vi "DAC8552 Example.vi"() -> ()   [LabVIEW 2020]
uses:
  <vilib>/MakerHub/LINX/Public/Peripherals/SPI/SPI CS Config.ctl
  <vilib>/MakerHub/LINX/Private/Type Defs/Peripherals/SPI/SPI CS Logic Level.ctl
  <vilib>/MakerHub/LINX/Private/Type Defs/Peripherals/SPI/SPI Configuration.ctl
  <vilib>/MakerHub/LINX/Private/Type Defs/Peripherals/SPI/SPI Bit Order.ctl
  <vilib>/MakerHub/LINX/Private/Type Defs/Peripherals/SPI/SPI Mode.ctl
  LINX-DAC8552/Power Down Mode.ctl
  LINX-DAC8552/Channel Select.ctl
  <vilib>/MakerHub/LINX/Public/Utilities/Open Local.vi
  LINX SPI/LINX SPI.lvclass
  <vilib>/MakerHub/LINX/LMH-LINX.lvlib
  LINX-DAC8552/LINX-DAC8552.lvclass
panel:
  in  "DAC B":dbl
  in  "DAC A":dbl
  in  "stop":bool
  out "Error Out":errorcluster
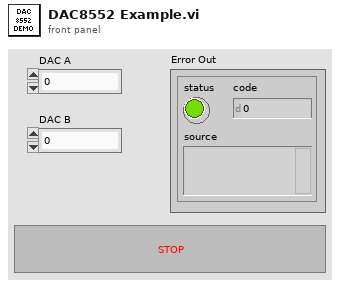
[diagram p1: front panel]
types:
  T1 = typedef "LINX-DAC8552.lvclass/Power Down Mode.ctl" = enum8{"On - Normal Operation", "Off - 1kOhm", "Off - 100kOhm", "Off - High Impedence"}
  T2 = typedef "LINX-DAC8552.lvclass/Channel Select.ctl" = enum8{"DAC A", "DAC B", "Both"}
  T3 = typedef "LMH-LINX.lvlib/SPI Configuration.ctl" = cluster{"Clock Frequency":u32, "Bit Order":T4, "SPI Mode":T5}
  T4 = typedef "LMH-LINX.lvlib/SPI Bit Order.ctl" = enum8{"LSb First", "MSb First"}
  T5 = typedef "LMH-LINX.lvlib/SPI Mode.ctl" = enum8{"Mode 0", "Mode 1", "Mode 2", "Mode 3"}
  T6 = typedef "LMH-LINX.lvlib/SPI CS Config.ctl" = cluster{"CS Channel":u8, "CS Logic Level":T7}
  T7 = typedef "LMH-LINX.lvlib/SPI CS Logic Level.ctl" = enum8{"Active Low", "Active High"}
  T8 = typedef "LMH-LINX.lvlib/LINX Ref.ctl" = cluster{"IO":T9, "Interface":T10, "LINX Device Config":T11}
  T9 = typedef "LMH-LINX.lvlib/Platform.ctl" = enum16{"Remote", "Local"}
  T10 = typedef "LMH-LINX.lvlib/Interface.ctl" = enum16{"Serial", "TCP"}
  T11 = typedef "LMH-LINX.lvlib/Device.lvlib/LINX Device Config.ctl" = cluster{"Interface":T10, "COM Port":refnum<visa-resource-name>, "TCP Configuration":T12, "Device Family":u8, "Device ID":u8, "Device Name":string, "TCP Ref":refnum<k5>, "Channels":T13}
  T12 = typedef "LMH-LINX.lvlib/Device.lvlib/TCP Config.ctl" = cluster{"IP Address":string, "Port":u16}
  T13 = typedef "LMH-LINX.lvlib/Channels.ctl" = cluster{"DI":u8[], "DO":u8[], "AI":u8[], "AO":u8[], "PWM":u8[], "QE":u8[], "UART":u8[], "I2C 2":u8[], "SPI":u8[], "CAN":u8[], "Servo":u8[], "AI Ref (V)":dbl, "AI Resolution (Bits)":u8, "AO Ref (V)":dbl, "AO Resolution (Bits)":u8}
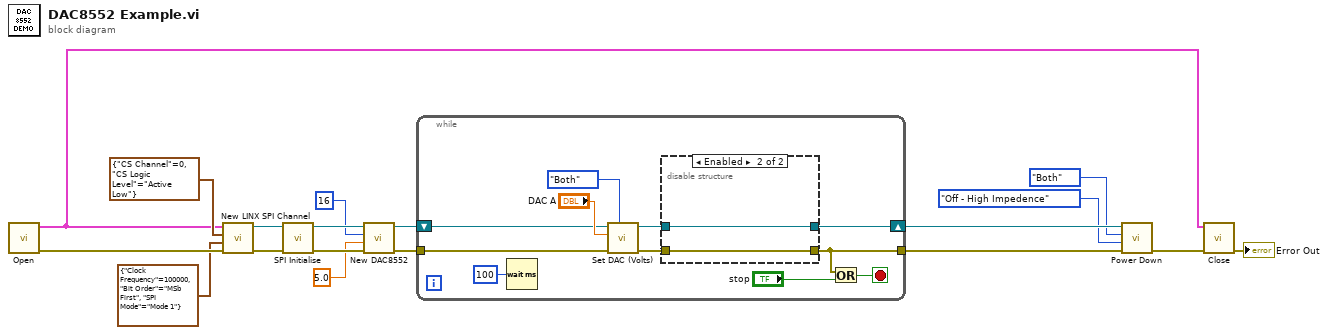
[diagram p0: block diagram]
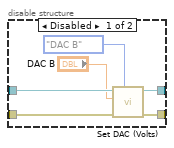
[diagram p2: hidden frame]
diagram:
  n1 = call-poly <vilib>:"Open.vi"() -> ("Error Out"=w17:errorcluster, "LINX Resource"=w13:T8)  [unwired: 9 in, 1 out]
  n2 = call "New LINX SPI Channel.vi"("error in (no error)"=w17, "SPI Configuration"=T3 {"Clock Frequency"=100000, "Bit Order"=enum."MSb First", "SPI Mode"=enum."Mode 1"}, "CS Configuration"=T6 {"CS Channel"=0, "CS Logic Level"=enum."Active Low"}, "LINX Resource"=w13) -> ("error out"=w14:errorcluster, "LINX SPI out"=w15:refnum<class "LINX SPI.lvclass">)  [unwired: 6 in]
  n3 = call-dynamic "SPI Initialise.vi"("error in (no error)"=w14, "LINX SPI in"=w15) -> ("error out"=w11:errorcluster, "LINX SPI out"=w10:refnum<class "LINX SPI.lvclass">)  [unwired: 8 in]
  n4 = call "New DAC8552.vi"("error in (no error)"=w11, "VRef (5V)"=5.0, "SPI CS Line"=u8 16, "SPI in"=w10) -> ("error out"=w6:errorcluster, "LINX-DAC8552 out"=w7:refnum<class "LINX-DAC8552.lvclass">)  [unwired: 6 in]
  n5 = while {
    tunnel: w6 -> [w26]
    shift-right: [w24] -> w3
    shift-left: w7 -> [w20]
    tunnel: [w25] -> w5
    stop <- w28 stop-if-true
    n6 = Wait (ms)(milliseconds to wait=u32 100) -> ()  [unwired: 1 out]
    n7 = call "Set DAC (Volts).vi"("Channel Select"=Channel_Select."Both", "error in (no error)"=w26, "DAC Output (V)"="DAC A", "DAC8552 in"=w20) -> ("error out"=w22:errorcluster, "DAC8552 out"=w23:refnum<class "LINX-DAC8552.lvclass">)  [unwired: 6 in]
    n8 = disable-structure shown="Enabled" {
      disable-tunnel: [w35 w36] -> w25
      disable-tunnel: [w34 w37] -> w24
      disable-tunnel: w23 -> [w33 w37]
      disable-tunnel: w22 -> [w32 w36]
      frame Disabled {
        n9 = call "Set DAC (Volts).vi"("Channel Select"=Channel_Select."DAC B", "error in (no error)"=w32, "DAC Output (V)"="DAC B", "DAC8552 in"=w33) -> ("error out"=w35:errorcluster, "DAC8552 out"=w34:refnum<class "LINX-DAC8552.lvclass">)  [unwired: 6 in]
      }
      frame Enabled {
      }
    }
    n10 = Or(x=w25, y="stop") -> (x .or. y?=w28:bool)
  }
  n11 = call "Power Down.vi"("error in (no error)"=w5, "Power Down Mode"=Power_Down_Mode."Off - High Impedence", "Channel Select"=Channel_Select."Both", "DAC8552 in"=w3) -> ("error out"=w4:errorcluster)  [unwired: 6 in, 1 out]
  n12 = call <vilib>:"Close.vi"("Error In"=w4, "LINX Resource"=w13) -> ("Error Out"=→"Error Out":errorcluster)  [unwired: 9 in]
